vi "OAT Demodulation Initial States.vi"(4 "filters":T1[](array[typedef]) {"coefficients" format="%.2f"}, 6 "CIC filter settings":T2={"interpolation/decimation factor"=2, "stages"=2, "lag"=1}, 7 "num of orders":i32, 8 "reset? (True)":bool=TRUE, 9 "imaginary state in":cluster{cluster{dbl[]}, cluster{dbl[]}[]}[](array[cluster]), 10 "real state in":cluster{cluster{dbl[]}, cluster{dbl[]}[]}[](array[cluster]), 11 "start phase in":dbl[](array[numeric]) format="%.2f") -> (1 "imaginary state out":cluster{cluster{dbl[]}, cluster{dbl[]}[]}[](array[cluster]), 2 "real state out":cluster{cluster{dbl[]}, cluster{dbl[]}[]}[](array[cluster]), 3 "start phase out":dbl[](array[numeric]) format="%.2f")   [LabVIEW 2017, in "SoundVib_Resampling.lvlib"]
uses:
  <vilib>/addons/Sound and Vibration/Order Analysis/Resample Order Tracking/SoundVib_Resampling.lvlib
  <vilib>/addons/_NISVFA/_Shared subVIs/Controls/OAT Decimation Filter.ctl
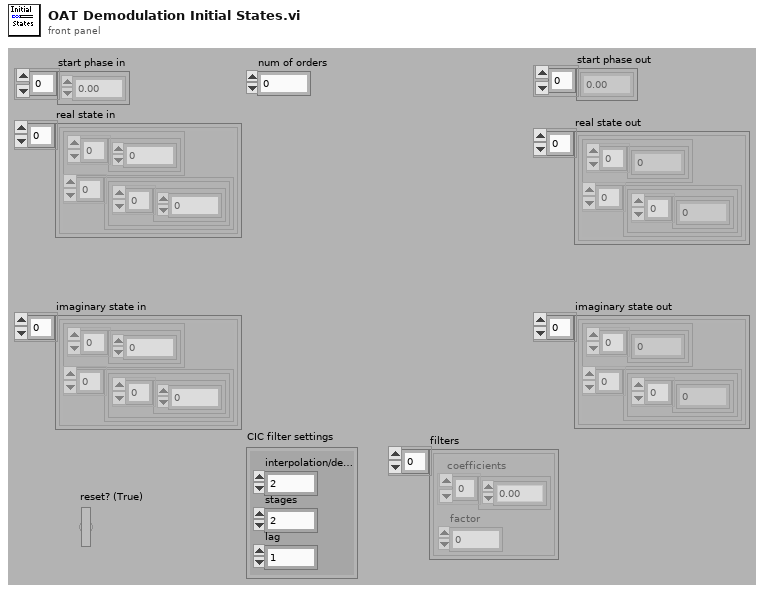
[diagram p1: front panel]
types:
  T1 = typedef "OAT Decimation Filter.ctl" = cluster{"coefficients":dbl[], "factor":i32}
  T2 = cluster{"interpolation/decimation factor":i32, "stages":i32, "lag":i32}
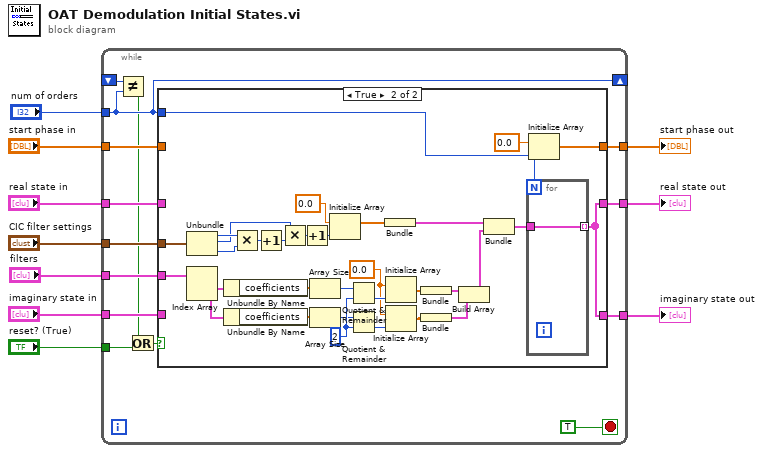
[diagram p0: block diagram]
diagram:
  n1 = while {
    tunnel: "reset? (True)" -> [w15]
    tunnel: "real state in" -> [w24]
    tunnel: [w23] -> w8
    tunnel: "start phase in" -> [w22]
    tunnel: "imaginary state in" -> [w21]
    tunnel: "CIC filter settings" -> [w20]
    tunnel: "filters" -> [w19]
    shift-right: [w16] -> _
    shift-left: _ -> [w17]
    tunnel: "num of orders" -> [w16]
    tunnel: [w12] -> w2
    tunnel: [w11] -> w1
    stop <- TRUE stop-if-true
    n2 = Not Equal?(x=w17, y=w16) -> (x != y?=w14:bool)
    n3 = Or(x=w14, y=w15) -> (x .or. y?=w13:bool)
    n4 = case shown="True" w13 {
      tunnel: w24 -> [w26 _]
      tunnel: w21 -> [w25 _]
      tunnel: [w27 w58] -> w23
      tunnel: w22 -> [w27 _]
      tunnel: w20 -> [_ w57]
      tunnel: w19 -> [_ w56]
      tunnel: w16 -> [_ w32]
      tunnel: [w26 w28] -> w12
      tunnel: [w25 w28] -> w11
      frame False {
      }
      frame True {
        w36 = 0.0 ("Element Data")
        w41 = 2 ("Element Data")
        n5 = Unbundle(w57) -> ("interpolation/decimation factor"=w52:i32, "stages"=w48:i32, "lag"=w51:i32)
        n6 = Index Array(array=w56) -> (element #1=w45:T1, element #2=w44:T1)  [unwired: 2 in]
        n7 = Unbundle By Name(w45) -> ("coefficients"=w43:dbl[])
        n8 = Unbundle By Name(w44) -> ("coefficients"=w42:dbl[])
        n9 = Multiply(x=w52, y=w51) -> (x*y=w50:i32)
        n10 = Increment(x=w50) -> (x+1=w49:i32)
        n11 = Multiply(x=w48, y=w49) -> (x*y=w47:i32)
        n12 = Increment(x=w47) -> (x+1=w46:i32)
        n13 = Array Size(array=w43) -> (size(s)=w40:i32)
        n14 = Array Size(array=w42) -> (size(s)=w39:i32)
        n15 = Initialize Array(0.0 ("Element Data"), w46) -> (w53:dbl[])
        n16 = Quotient & Remainder(x=w40, y=w41) -> (floor(x/y)=w38:i32)  [unwired: 1 out]
        n17 = Quotient & Remainder(x=w39, y=w41) -> (floor(x/y)=w37:i32)  [unwired: 1 out]
        n18 = Bundle(w53) -> (w33:cluster{dbl[]})  [unwired: 1 in]
        n19 = Initialize Array(w36, w38) -> (w34:dbl[])
        n20 = Initialize Array(w36, w37) -> (w35:dbl[])
        n21 = Bundle(w34) -> (w31:cluster{dbl[]})  [unwired: 1 in]
        n22 = Bundle(w35) -> (w30:cluster{dbl[]})  [unwired: 1 in]
        n23 = Build Array(w31, w30) -> (w29:cluster{dbl[]}[])
        n24 = Bundle(w33, w29) -> (w55:cluster{cluster{dbl[]}, cluster{dbl[]}[]})  [unwired: 1 in]
        n25 = for {
          N: w32 -> [_]
          tunnel: w55 -> [w60]
          tunnel: [w60] -> w28 mode=indexing
        }
        n26 = Initialize Array(0.0 ("Element Data"), w32) -> (w58:dbl[])
      }
    }
  }
  "start phase out" <- w8
  "real state out" <- w2
  "imaginary state out" <- w1
